vi "Run Action_Do.vi"(8 "error in (no error)":errorcluster, 10 "Project Builder in":refnum<class "Project Builder.lvclass">, 11 "Caraya Unit Test":refnum<class "Caraya Test.lvclass">) -> (0 "error out":errorcluster, 1 "Success?":bool, 3 "Report":refnum<class "Report Data.lvclass">)   [LabVIEW 2019, in "ProjectBuilder.lvlib" / "Caraya Test.lvclass"]
doc: "Run the action associated with the 'Project Action'-class.\n\nThis implementation runs a project pased Caraya-test using the settings from the private data."
uses:
  Caraya Test.lvclass
  C:/WS/prev/LV32.2019..ProjectBuilder/Class/Project Action/Project Action.lvclass
  Data/Report Data/Report Data.lvclass
  Project Builder/Project Builder.lvclass
  Project Action/Project Action.lvclass/Project Action.ctl
  Caraya Test.lvclass/Caraya Test.ctl
  Caraya Status Data/Caraya Status Data.lvclass/Caraya Status Data.ctl
  Caraya Status Data/Caraya Status Data.lvclass
  C:/WS/prev/LV32.2019..ProjectBuilder/Class/Data/Report Data/Report Data.lvclass
  Project Action/Project Action.lvclass
  ProjectBuilder.lvlib
  PPL/Caraya.lvlibp
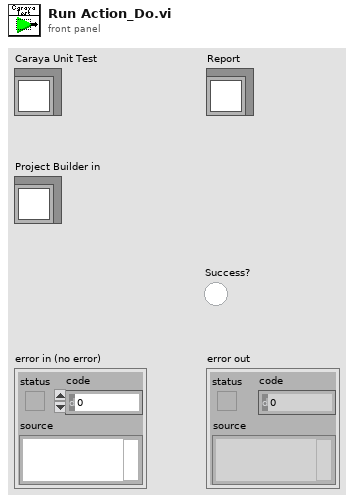
[diagram p1: front panel]
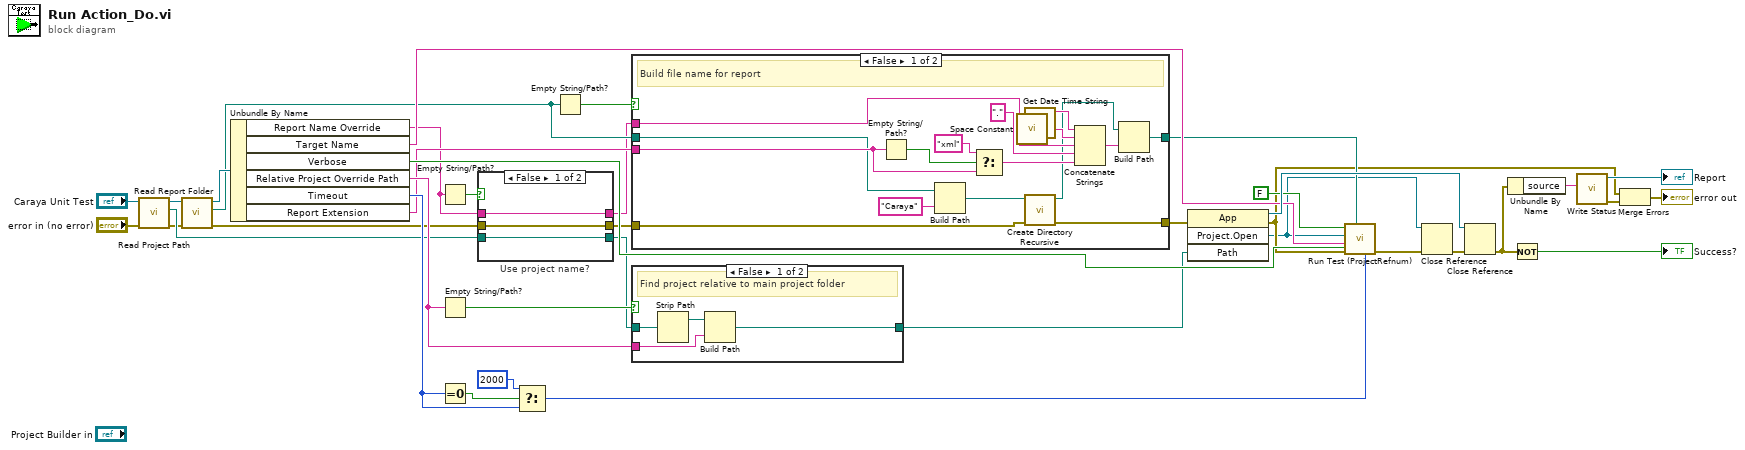
[diagram p0: block diagram]
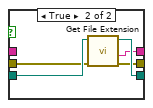
[diagram p2: hidden frame]
diagram:
  n1 = call "Read Project Path.vi"("error in (no error)"="error in (no error)", "Project Action in"="Caraya Unit Test") -> ("error out"=w18:errorcluster, "Project Path"=w23:path, "Project Action out"=w20:refnum<class "Caraya Test.lvclass">)  [unwired: 7 in]
  n2 = call "Read Report Folder.vi"("error in (no error)"=w18, "Project Action in"=w20) -> ("error out"=w17:errorcluster, "Report Folder"=w14:path, "Project Action out"=w19:refnum<class "Caraya Test.lvclass">)  [unwired: 7 in]
  n3 = Unbundle By Name(w19) -> ("Report Name Override"=w9:string, "Target Name"=w33:string, "Verbose"=w32:bool, "Relative Project Override Path"=w29:string, "Timeout"=w26:i32, "Report Extension"=w21:string)
  n4 = Empty String/Path?(string/path=w9) -> (empty?=w10:bool)
  n5 = Empty String/Path?(string/path=w29) -> (empty?=w31:bool)
  n6 = Equal To 0?(x=w26) -> (x = 0?=w27:bool)
  n7 = case "Use project name?" shown="False" w10 {
    tunnel: w23 -> [w41 w46]
    tunnel: [w41 w45] -> w22
    tunnel: [w40 w44] -> w1
    tunnel: w17 -> [w39 w43]
    tunnel: [w39 w42] -> w13
    tunnel: w9 -> [w40 _]
    frame False {
    }
    frame True {
      n8 = call <vilib>:"Get File Extension.vi"("error in (no error)"=w43, "file"=w46) -> ("error out"=w42:errorcluster, "filename without extension"=w44:string, "dup file"=w45:path)  [unwired: 5 in, 2 out]
    }
  }
  n9 = Select(t=2000, s=w27, f=w26) -> (s? t:f=w24:i32)
  n10 = Empty String/Path?(string/path=w14) -> (empty?=w16:bool)
  n11 = case shown="False" w16 {
    tunnel: w1 -> [w60 _]
    tunnel: w21 -> [w57 _]
    tunnel: [w50 w64] -> w15
    tunnel: w14 -> [w48 w64]
    tunnel: w13 -> [w54 w63]
    tunnel: [w53 w63] -> w12
    frame False {
      # "Build file name for report"
      n12 = Empty String/Path?(string/path=w57) -> (empty?=w58:bool)
      n13 = Build Path(base path=w48, name or relative path="Caraya" ("t")) -> (appended path=w49:path)
      n14 = Select(t="xml", s=w58, f=w57) -> (s? t:f=w55:string)
      n15 = call <vilib>:"Space Constant.vi"() -> ("String"=w61:string)
      n16 = call "Get Date Time String.vi"() -> ("Time String"=w62:string)  [unwired: 11 in]
      n17 = call <vilib>:"Create Directory Recursive.vi"("error in (no error)"=w54, "directory"=w49) -> ("error out"=w53:errorcluster, "directory copy"=w52:path)  [unwired: 3 in, 1 out]
      n18 = Concatenate Strings(w62, w61, w60, "." ("string"), w55) -> (w51:string)
      n19 = Build Path(base path=w52, name or relative path=w51) -> (appended path=w50:path)
    }
    frame True {
      # "No report"
    }
  }
  n20 = case shown="False" w31 {
    tunnel: [w65 w69] -> w30
    tunnel: w22 -> [w68 w69]
    tunnel: w29 -> [w66 _]
    frame False {
      # "Find project relative to main project folder"
      n21 = Strip Path(path=w68) -> (stripped path=w67:path)  [unwired: 1 out]
      n22 = Build Path(base path=w67, name or relative path=w66) -> (appended path=w65:path)
    }
    frame True {
      # "No override"
    }
  }
  n23 = invoke class="App" method="Project.Open"(error in=w12, "Path"=w30) -> (reference out=w38:refnum<vi>, error out=w6:errorcluster, "Project:Open"=w2:refnum<vi>)  [unwired: 2 in, 1 out]
  n24 = call "Run Test (ProjectRefnum).vi"("timeout (2000 ms)"=w24, "Verbose"=w32, "Report Path"=w15, "error in"=w6, "Virtual Folder (My Computer)"=w33, "Project Refnum"=w2, "Interactive (T)"=FALSE) -> ("error out"=w4:errorcluster)  [unwired: 3 in, 1 out]
  n25 = Close Reference(reference=w2, error in (no error)=w4) -> (error out=w3:errorcluster)
  n26 = Close Reference(reference=w38, error in (no error)=w3) -> (error out=w28:errorcluster)
  n27 = Unbundle By Name(w28) -> ("source"=w8:string)
  n28 = Not(x=w28) -> (.not. x?=→"Success?":bool)
  n29 = call "Write Status.vi"("Status"=w8) -> ("error out"=w7:errorcluster, "Caraya Status Data out"=→"Report":refnum<class "Caraya Status Data.lvclass">)  [unwired: 9 in]
  n30 = Merge Errors(w6, w7) -> (→"error out":errorcluster)
